vi "ReadTouchScreenData.vi"(10 "Interrupt data":u8[](array[numeric])) -> (0 "Y Pixel":u32, 1 "X Pixel":u32, 2 "Measured Y":dbl, 3 "Measured X":dbl)   [LabVIEW 2015]
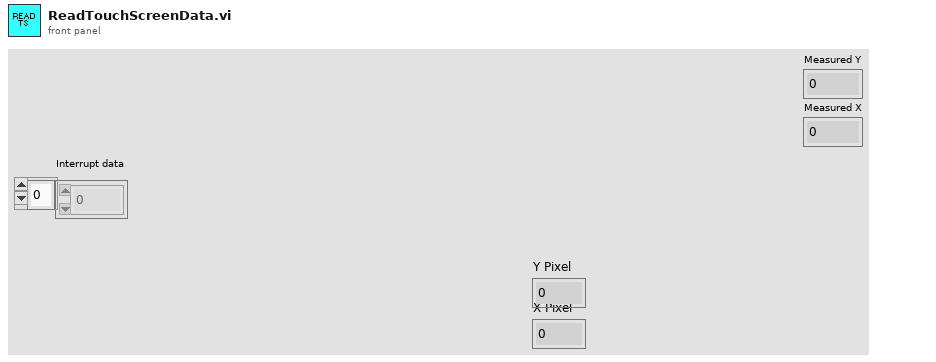
[diagram p1: front panel]
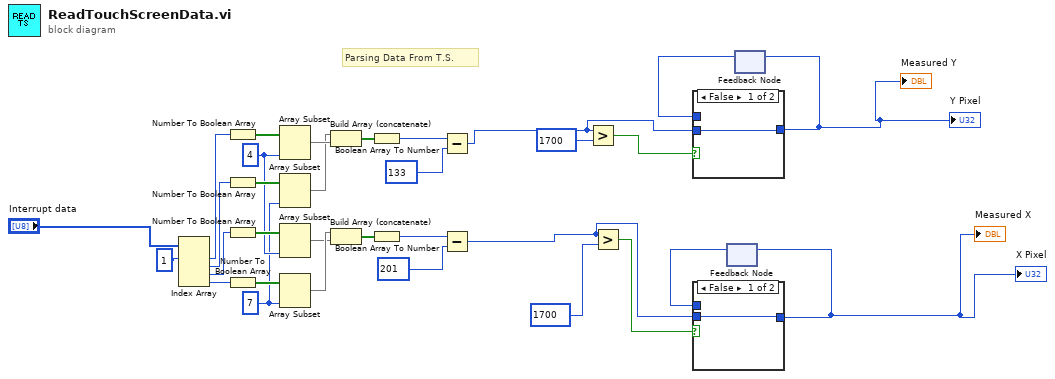
[diagram p0: block diagram]
diagram:
  w16 = 7 ("length")
  w17 = 4 ("length")
  # "Parsing Data From T.S."
  n1 = Index Array(array="Interrupt data", index #1=1 ("index")) -> (element #1=w20:u8, element #2=w19:u8, element #3=w29:u8, element #4=w30:u8)  [unwired: 3 in]
  n2 = Number To Boolean Array(number=w20) -> (Boolean array=w21:bool[])
  n3 = Number To Boolean Array(number=w19) -> (Boolean array=w22:bool[])
  n4 = Number To Boolean Array(number=w29) -> (Boolean array=w31:bool[])
  n5 = Number To Boolean Array(number=w30) -> (Boolean array=w32:bool[])
  n6 = Array Subset(array=w21, length=w17) -> (w24:bool[])  [unwired: 1 in]
  n7 = Array Subset(array=w22, length=w16) -> (w23:bool[])  [unwired: 1 in]
  n8 = Array Subset(array=w31, length=w17) -> (w27:bool[])  [unwired: 1 in]
  n9 = Array Subset(array=w32, length=w16) -> (w28:bool[])  [unwired: 1 in]
  n10 = Build Array (concatenate)(w23, w24) -> (w25:bool[])
  n11 = Build Array (concatenate)(w28, w27) -> (w26:bool[])
  n12 = Boolean Array To Number(Boolean array=w25) -> (number=w15:u32)
  n13 = Boolean Array To Number(Boolean array=w26) -> (number=w13:u32)
  n14 = Subtract(x=w15, y=u32 133) -> (x-y=w8:u32)
  n15 = Subtract(x=w13, y=u32 201) -> (x-y=w6:u32)
  n16 = Greater?(x=w8, y=u32 1700) -> (0:w10:bool)
  n17 = Greater?(x=w6, y=u32 1700) -> (0:w7:bool)
  n18 = feedback #1() -> (w11:u32)  [unwired: 1 in]
  n19 = case shown="False" w7 {
    tunnel: [w33 w34] -> w2
    tunnel: w11 -> [_ w34]
    tunnel: w6 -> [w33 _]
    frame False {
    }
    frame True {
    }
  }
  "X Pixel" <- w2
  "Measured X" <- w2
  n20 = feedback-in #1(w2) -> ()
  n21 = feedback #2() -> (w9:u32)  [unwired: 1 in]
  n22 = case shown="False" w10 {
    tunnel: [w35 w36] -> w1
    tunnel: w9 -> [_ w36]
    tunnel: w8 -> [w35 _]
    frame False {
    }
    frame True {
    }
  }
  "Y Pixel" <- w1
  "Measured Y" <- w1
  n23 = feedback-in #2(w1) -> ()
